vi "Do.vi"(8 "error in (no error)":errorcluster, 10 "Actor in":refnum<class "Actor.lvclass">, 11 "DNL_Message Template":refnum<class "Write Message Stream_Msg.lvclass">) -> (0 "error out":errorcluster, 2 "Actor out":refnum<class "Actor.lvclass">)   [LabVIEW 2023, in "Write Message Stream_Msg.lvclass"]
doc: "This VI delivers the message to the actor by calling the appropriate method(s) on the actor."
uses:
  Write Message Stream_Msg.lvclass
  <vilib>/ActorFramework/Actor/Actor.lvclass
  Write Message Stream_Msg.lvclass/Write Message Stream_Msg.ctl
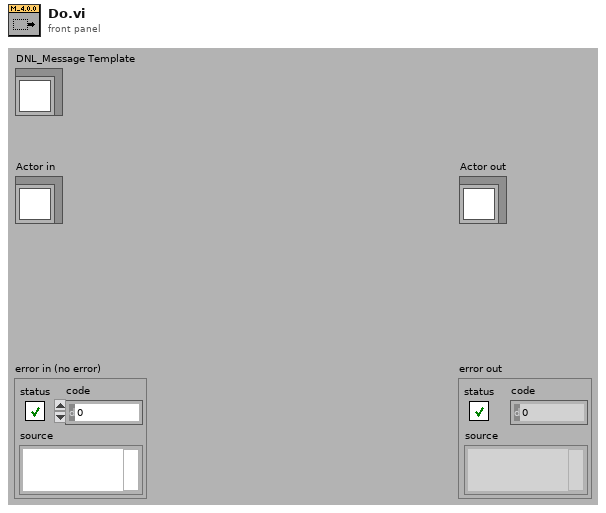
[diagram p1: front panel]
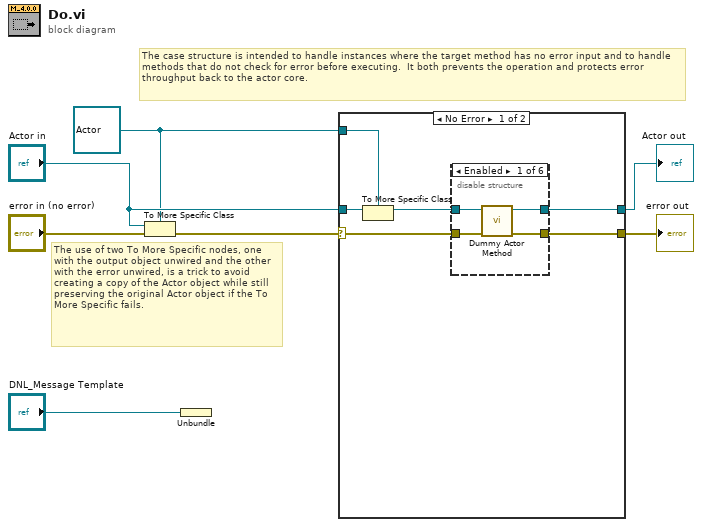
[diagram p0: block diagram]
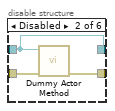
[diagram p2: hidden frame]
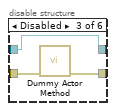
[diagram p3: hidden frame]
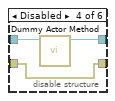
[diagram p4: hidden frame]
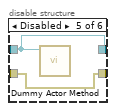
[diagram p5: hidden frame]
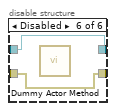
[diagram p6: hidden frame]
diagram:
  w1 = refnum<class "Actor.lvclass"> refnum ("Actor in")
  # "The use of two To More Specific nodes, one with the output object unwired and the other with the error unwired, is a trick to avoid creating a copy of the Actor object while still preserving the original Actor object if the To More Specific fails."
  # "The case structure is intended to handle instances where the target method has no error input and to handle methods that do not check for error before executing.  It both prevents the operation and protects error throughput back to the actor core."
  n1 = To More Specific Class(target class=w1, reference="Actor in", error in="error in (no error)") -> (error out=w5:errorcluster)  [unwired: 1 out]
  n2 = Unbundle("DNL_Message Template") -> ()  [unwired: 1 out]
  n3 = case shown="No Error" w5 {
    selector: w5 -> [w11 w32]
    tunnel: [w13 w32] -> w4
    tunnel: [w12 w31] -> w3
    tunnel: "Actor in" -> [w10 w31]
    tunnel: w1 -> [w9 _]
    frame No Error {
      n4 = To More Specific Class(target class=w9, reference=w10) -> (specific class reference=w8:refnum<class "Actor.lvclass">)  [unwired: 1 in, 1 out]
      n5 = disable-structure shown="Enabled" {
        disable-tunnel: [w17 w20 w23 w25 w28 w30] -> w13
        disable-tunnel: [w16 w18 w21 w26 w27 w29] -> w12
        disable-tunnel: w11 -> [w15 w19 w22 w25 w28 w30]
        disable-tunnel: w8 -> [w14 w18 w21 w24 w27 w29]
        frame Enabled {
          n6 = call <resource>:"Dummy Actor Method.vi"("error in (no error)"=w15, "Actor in"=w14) -> ("error out"=w17:errorcluster, "Actor out"=w16:refnum<class "Actor.lvclass">)  [unwired: 8 in]
        }
        frame Disabled {
          n7 = call <resource>:"Dummy Actor Method.vi"("error in (no error)"=w19, "Actor in"=w18) -> ("error out"=w20:errorcluster)  [unwired: 8 in, 1 out]
        }
        frame Disabled {
          n8 = call <resource>:"Dummy Actor Method.vi"("error in (no error)"=w22) -> ("error out"=w23:errorcluster)  [unwired: 9 in, 1 out]
        }
        frame Disabled {
          n9 = call <resource>:"Dummy Actor Method.vi"("Actor in"=w24) -> ("Actor out"=w26:refnum<class "Actor.lvclass">)  [unwired: 9 in, 1 out]
        }
        frame Disabled {
          n10 = call <resource>:"Dummy Actor Method.vi"("Actor in"=w27) -> ()  [unwired: 9 in, 2 out]
        }
        frame Disabled {
          n11 = call <resource>:"Dummy Actor Method.vi"() -> ()  [unwired: 10 in, 2 out]
        }
      }
    }
    frame Error {
      # "If type check fails, pass the original object out again."
    }
  }
  "error out" <- w4
  "Actor out" <- w3
